vi "XLP80_Datalog_CreateHeader.vi"() -> (3 "Header":string)   [LabVIEW 2021]
uses:
  XLP80_FGlob/XLP80_FGLob_TDefEnumCalcAnalogItems.ctl
  XLP80_Globals/Globals_Settings_XLP80.vi
panel:
  in  "CalcReal Item":T1
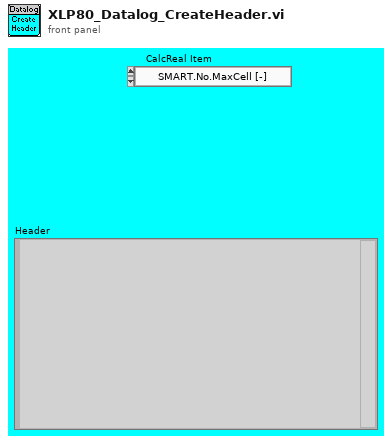
[diagram p1: front panel]
types:
  T1 = typedef "XLP80_FGLob_TDefEnumCalcAnalogItems.ctl" = enum8{"SMART.No.MaxCell [-]", "SMART.No.MinCell [-]", "SMART.U.S.AveCell [V]", "SMART.U.S.CVM [V]", "SMART.U.S.MaxCell [V]", "SMART.U.S.MinCell [V]"}
  T2 = typedef "XLP80_Datalog_TypeDefEnumLogselect.ctl" = enum16{"SMART.No.MaxCell [-]", "SMART.No.MinCell [-]", "SMART.U.S.AveCell [V]", "SMART.U.S.CVM [V]", "SMART.U.S.MaxCell [V]", "SMART.U.S.MinCell [V]"}
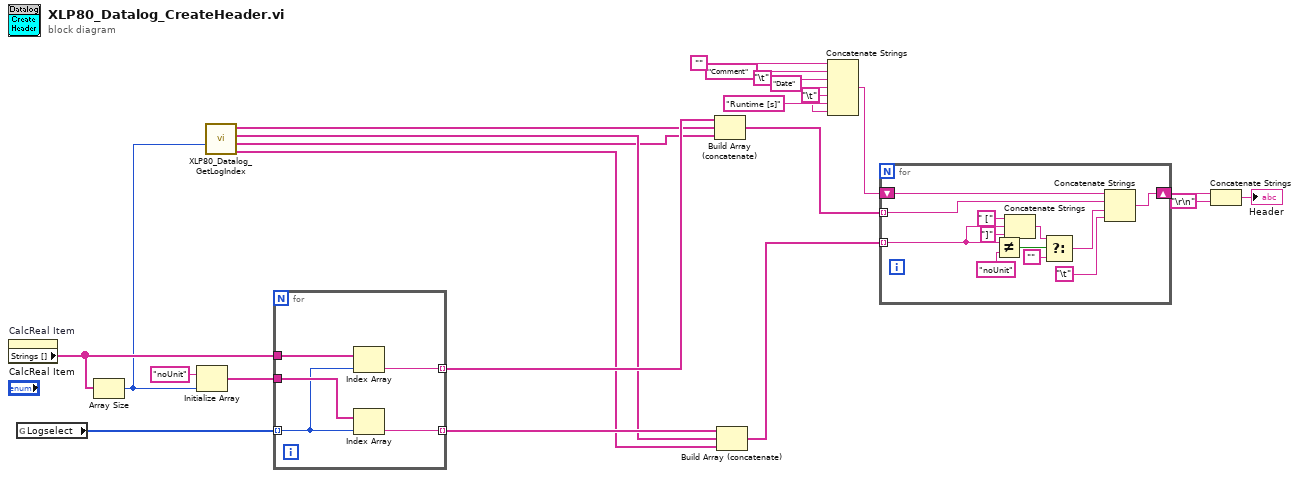
[diagram p0: block diagram]
diagram:
  w14 = "\t" ("Substring")
  n1 = property on="CalcReal Item" class="Enum (strict)"() -> ("Strings []"=w13:string[])  [unwired: 2 in, 2 out]
  n2 = global read "Globals_Settings_XLP80.vi" "Logselect"() -> (w4:T2[])
  n3 = Array Size(array=w13) -> (size(s)=w9:i32)
  n4 = Initialize Array("noUnit", w9) -> (w11:string[])
  n5 = call "XLP80_Datalog_GetLogIndex.vi"("CalcValueSize"=w9) -> ("Unit Write"=w5:string[], "Name Write"=w6:string[], "Unit Read"=w7:string[], "Name Read"=w8:string[])  [unwired: 6 in, 1 out]
  n6 = for {
    tunnel: w4 -> [w25] mode=indexing
    tunnel: w13 -> [w28]
    tunnel: [w27] -> w12 mode=indexing
    tunnel: w11 -> [w26]
    tunnel: [w24] -> w10 mode=indexing
    n7 = Index Array(array=w28, index=w25) -> (element=w27:string)
    n8 = Index Array(array=w26, index=w25) -> (element=w24:string)
  }
  n9 = Build Array (concatenate)(w12, w8, w6) -> (w16:string[])
  n10 = Build Array (concatenate)(w10, w7, w5) -> (w15:string[])
  n11 = Concatenate Strings("" ("Substring"), "Comment" ("Substring"), "\t" ("Substring"), "Date" ("Substring"), w14, "Runtime [s]" ("Substring"), w14) -> (w17:string)
  n12 = for {
    shift-right: [w40] -> w3
    shift-left: w17 -> [w39]
    tunnel: w16 -> [w31] mode=indexing
    tunnel: w15 -> [w30] mode=indexing
    n13 = Not Equal?(x=w30, y="noUnit") -> (x != y?=w34:bool)
    n14 = Concatenate Strings(" [" ("string"), w30, "]" ("string")) -> (w38:string)
    n15 = Select(t=w38, s=w34, f="") -> (s? t:f=w32:string)
    n16 = Concatenate Strings(w39, w31, w32, "\t") -> (w40:string)
  }
  n17 = Concatenate Strings(w3, "\r\n") -> (→"Header":string)
